vi "Get_Process_Details.vi"(0 "Process_Data":string[](array[string])) -> (4 "Needs":string[][](array[string]))   [LabVIEW 2023]
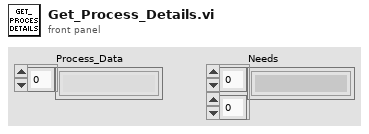
[diagram p1: front panel]
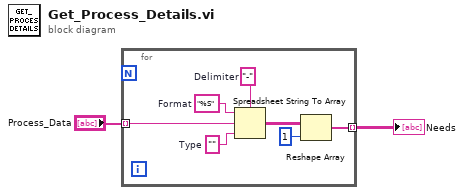
[diagram p0: block diagram]
diagram:
  n1 = for {
    tunnel: "Process_Data" -> [w9] mode=indexing
    tunnel: [w4] -> w1 mode=indexing
    w3 = "%S"  # Format
    w7 = ""  # Type
    w8 = "-"  # Delimiter
    n2 = Spreadsheet String To Array(delimiter (Tab)=w8, format string=w3, spreadsheet string=w9, array type (2D Dbl)=w7) -> (array=w6:string[][])
    n3 = Reshape Array(w6, 1 ("dimension size")) -> (w4:string[])
  }
  "Needs" <- w1
